vi "MPU digital to analog data.vi"(5 "Gyro FSR":T4, 6 "Mag bit depth":T3=enum."16bit", 7 "Accel FSR":T5, 8 "Error In":errorcluster, 10 "Digital MPU data":T2) -> (0 "Error Out":errorcluster, 2 "Analog MPU data":T1)   [LabVIEW 2016]
uses:
  Typedef/Accel FSR.ctl
  Typedef/Gyro FSR.ctl
  Typedef/Mag bit depth.ctl
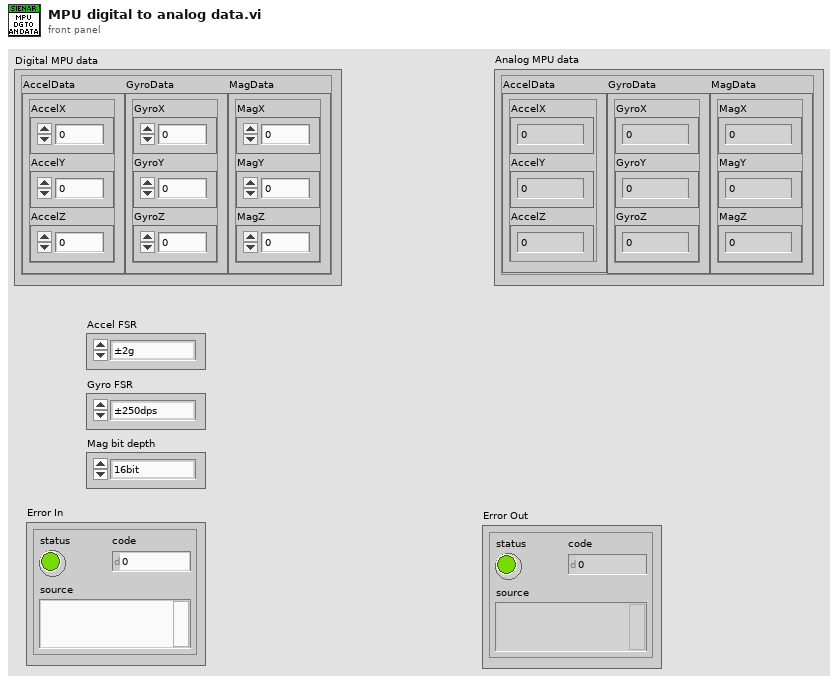
[diagram p1: front panel]
types:
  T1 = cluster{"AccelData":cluster{"AccelX":dbl, "AccelY":dbl, "AccelZ":dbl}, "GyroData":cluster{"GyroX":dbl, "GyroY":dbl, "GyroZ":dbl}, "MagData":cluster{"MagX":dbl, "MagY":dbl, "MagZ":dbl}}
  T2 = cluster{"AccelData":cluster{"AccelX":i16, "AccelY":i16, "AccelZ":i16}, "GyroData":cluster{"GyroX":i16, "GyroY":i16, "GyroZ":i16}, "MagData":cluster{"MagX":i16, "MagY":i16, "MagZ":i16}}
  T3 = typedef "Mag bit depth.ctl" = enum16{"14bit", "16bit"}
  T4 = typedef "Gyro FSR.ctl" = enum16{"±250dps", "±500dps", "±1000dps", "±2000dps"}
  T5 = typedef "Accel FSR.ctl" = enum16{"±2g", "±4g", "±8g", "±16g"}
  T6 = cluster{"AccelX":i16, "AccelY":i16, "AccelZ":i16}
  T7 = cluster{cluster{"[0]":dbl, "[1]":dbl, "[2]":dbl}, cluster{"[0]":dbl, "[1]":dbl, "[2]":dbl}, cluster{"[0]":dbl, "[1]":dbl, "[2]":dbl}}
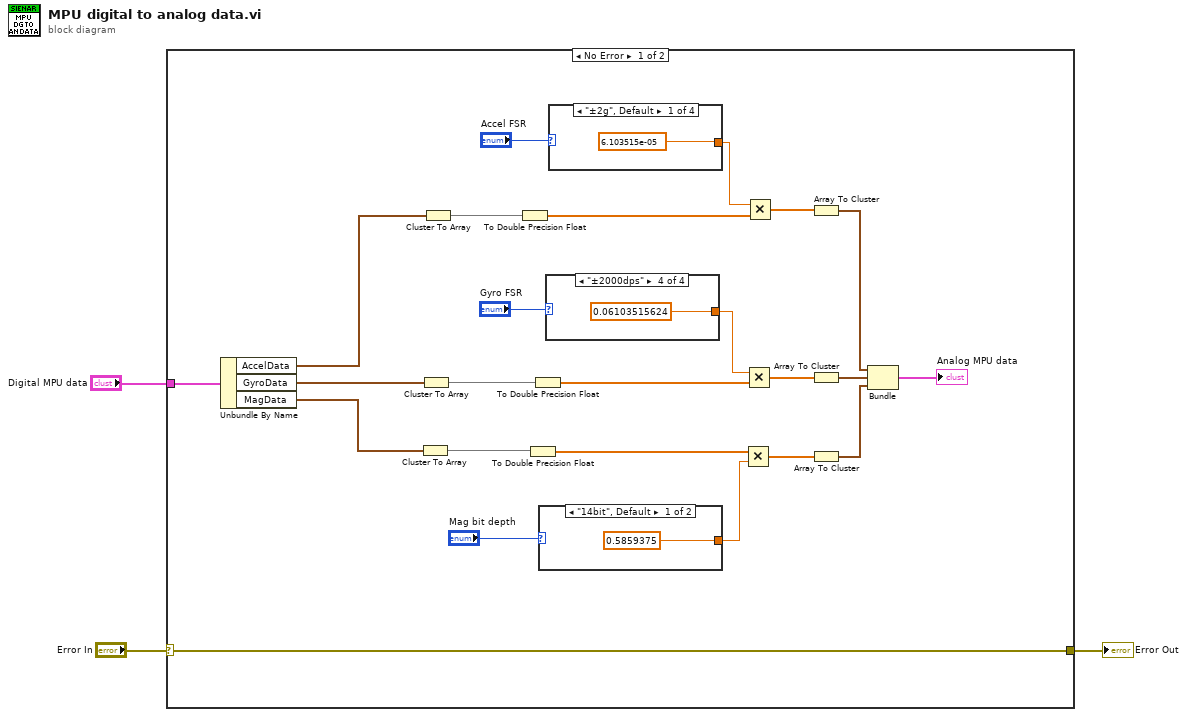
[diagram p0: block diagram]
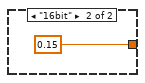
[diagram p2: hidden frame]
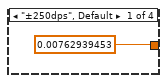
[diagram p3: hidden frame]
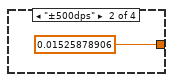
[diagram p4: hidden frame]
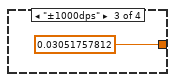
[diagram p5: hidden frame]
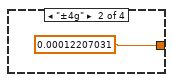
[diagram p6: hidden frame]
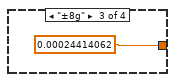
[diagram p7: hidden frame]
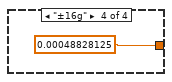
[diagram p8: hidden frame]
diagram:
  n1 = case shown="No Error" "Error In" {
    selector: "Error In" -> [w20 w38]
    tunnel: [w20 w38] -> w2
    tunnel: "Digital MPU data" -> [w11 _]
    frame No Error {
      n2 = Unbundle By Name(w11) -> ("AccelData"=w10:T6, "GyroData"=w9:cluster{"GyroX":i16, "GyroY":i16, "GyroZ":i16}, "MagData"=w8:cluster{"MagX":i16, "MagY":i16, "MagZ":i16})
      n3 = Cluster To Array(cluster=w8) -> (array=w12:i16[])
      n4 = Cluster To Array(cluster=w9) -> (array=w13:i16[])
      n5 = Cluster To Array(cluster=w10) -> (array=w14:i16[])
      n6 = To Double Precision Float(number=w14) -> (double precision float=w27:dbl[])
      n7 = To Double Precision Float(number=w12) -> (double precision float=w18:dbl[])
      n8 = To Double Precision Float(number=w13) -> (double precision float=w26:dbl[])
      n9 = case shown="\"14bit\", Default" "Mag bit depth" {
        tunnel: [0.5859375 0.15] -> w16
        frame "14bit", Default {
        }
        frame "16bit" {
        }
      }
      n10 = case shown="\"±2000dps\"" "Gyro FSR" {
        tunnel: [0.00762939453 0.01525878906 0.03051757812 0.06103515624] -> w21
        frame "±250dps", Default {
        }
        frame "±500dps" {
        }
        frame "±1000dps" {
        }
        frame "±2000dps" {
        }
      }
      n11 = case shown="\"±2g\", Default" "Accel FSR" {
        tunnel: [6.103515e-05 0.00012207031 0.00024414062 0.00048828125] -> w23
        frame "±2g", Default {
        }
        frame "±4g" {
        }
        frame "±8g" {
        }
        frame "±16g" {
        }
      }
      n12 = Multiply(x=w18, y=w16) -> (x*y=w19:dbl[])
      n13 = Multiply(x=w21, y=w26) -> (x*y=w25:dbl[])
      n14 = Multiply(x=w23, y=w27) -> (x*y=w15:dbl[])
      n15 = Array To Cluster(array=w15) -> (cluster=w7:cluster{"[0]":dbl, "[1]":dbl, "[2]":dbl})
      n16 = Array To Cluster(array=w25) -> (cluster=w6:cluster{"[0]":dbl, "[1]":dbl, "[2]":dbl})
      n17 = Array To Cluster(array=w19) -> (cluster=w5:cluster{"[0]":dbl, "[1]":dbl, "[2]":dbl})
      n18 = Bundle(w7, w6, w5) -> (→"Analog MPU data":T7)  [unwired: 1 in]
    }
    frame Error {
    }
  }
  "Error Out" <- w2
